vi "Recreate Client.vi"(8 "error in":errorcluster, 10 "cluster id":string, 11 "grpc client id in":T1) -> (0 "error out":errorcluster, 3 "grpc client id out":T1)   [LabVIEW 2020, in "NI Discovery V1 Client.lvlib"]
uses:
  NI Discovery V1 Client.lvlib
  <vilib>/gRPC/LabVIEW gRPC Library/Shared/grpcId.ctl
  gRPC/Generated APIs/ni/measurementlink/discovery/v1/ni.measurementlink.discovery.v1.api.lvlib
  <vilib>/gRPC/LabVIEW gRPC Library/grpc-lvsupport-release.lvlib
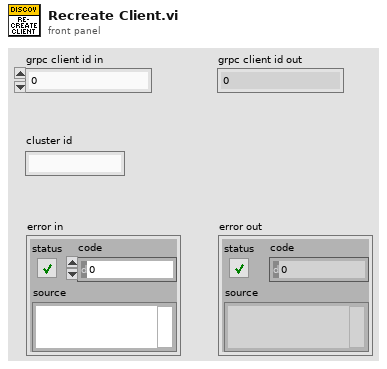
[diagram p1: front panel]
types:
  T1 = typedef "grpc-lvsupport-release.lvlib/grpcId.ctl" = u64
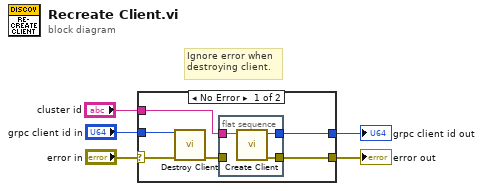
[diagram p0: block diagram]
diagram:
  # "Ignore error when\ndestroying client."
  n1 = case shown="No Error" "error in" {
    selector: "error in" -> [w11 w15]
    tunnel: [w10 w15] -> w4
    tunnel: [w9 _] -> w3
    tunnel: "grpc client id in" -> [w8 _]
    tunnel: "cluster id" -> [w6 _]
    frame No Error {
      n2 = call "Destroy Client.vi"("error in"=w11, "gRPC ID"=w8) -> ("error out"=w7:errorcluster)  [unwired: 9 in]
      n3 = flat-sequence {
        tunnel: [w14] -> w10
        tunnel: [w13] -> w9
        tunnel: w7 -> [_]
        tunnel: w6 -> [w12]
        frame #0 {
          n4 = call "Create Client.vi"("cluster id"=w12) -> ("error out"=w14:errorcluster, "grpc client id"=w13:T1)  [unwired: 9 in]
        }
      }
    }
    frame Error {
    }
  }
  "error out" <- w4
  "grpc client id out" <- w3
